vi "Start.vi"(8 "error in":errorcluster, 11 "Rx UDP Execution Unit in":refnum<class "Rx UDP Execution Unit.lvclass">) -> (0 "error out":errorcluster, 3 "Rx UDP Execution Unit out":refnum<class "Rx UDP Execution Unit.lvclass">)   [LabVIEW 2020, in "AIM ARINC 664 Engine.lvlib" / "Implementation.lvlib" / "Rx UDP Execution Unit.lvclass"]
uses:
  Rx UDP Execution Unit.lvclass
  Rx UDP Execution Unit.lvclass/Rx UDP Execution Unit.ctl
  <instrlib>/AIM GmbH/_AIM 664/bsp/Fdx Start (Rx).vi
  <instrlib>/AIM GmbH/_AIM 664/AIM664LV.lvlib
  <vilib>/Utility/SystemLogging/NI_SystemLogging.lvlib
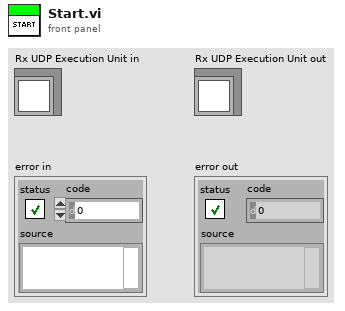
[diagram p1: front panel]
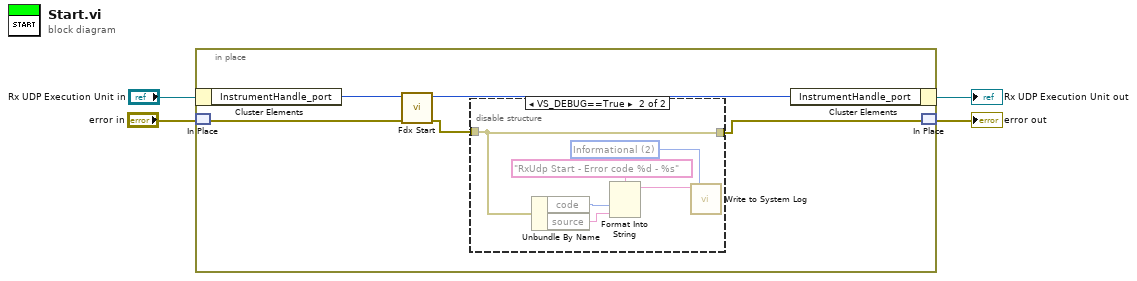
[diagram p0: block diagram]
diagram:
  n1 = in-place {
    n2 = in-place-cluster #1("Rx UDP Execution Unit in") -> ("InstrumentHandle_port"=w8:u32)
    n3 = in-place-match #2("error in") -> (w9:errorcluster)
    n4 = call-poly <instrlib>:"Fdx Start.vi"("error in"=w9, "InstrumentHandle_port in"=w8) -> ("error out"=w6:errorcluster, "InstrumentHandle_port out"=w7:u32)  [unwired: 8 in]
    n5 = disable-structure shown="VS_DEBUG==True" {
      disable-tunnel: w6 -> [w10 w11]
      disable-tunnel: [w10 w11] -> w5
      frame condition #0 (active) {
      }
      frame condition #1 {
        w14 = 2 items=["Error", "Warning", "Informational"] ("severity")
        n6 = Unbundle By Name(w11) -> ("code"=w13:i32, "source"=w12:string)
        n7 = Format Into String(format string="RxUdp Start - Error code %d - %s", w13, w12) -> (resulting string=w15:string)  [unwired: 2 in, 1 out]
        n8 = call <vilib>:"Write to System Log.vi"("severity"=w14, "message"=w15) -> ()  [unwired: 9 in, 1 out]
      }
    }
    n9 = in-place-cluster #1("InstrumentHandle_port"=w7) -> (→"Rx UDP Execution Unit out":refnum<class "Rx UDP Execution Unit.lvclass">)
    n10 = in-place-match #2(w5) -> (→"error out":errorcluster)
  }
